vi "Disable.vi"(8 "error in (no error)":errorcluster {"code" format="%.0x"}, 11 "instrument handle":refnum<k15>) -> (0 "error out":errorcluster {"code" format="%.0x"}, 3 "instrument handle out":refnum<k15>)   [LabVIEW 2021, in "Keysight XSAnVMA.lvlib"]
doc: "Quickly places the instrument in a state where it has no, or minimal, effect on the external system to which it is connected. This state is not necessarily a known state."
uses:
  <instrlib>/Keysight XSAnVMA/Keysight XSAnVMA.lvlib
  KtXSAnVMA_64.dll
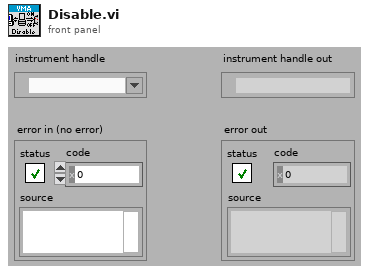
[diagram p1: front panel]
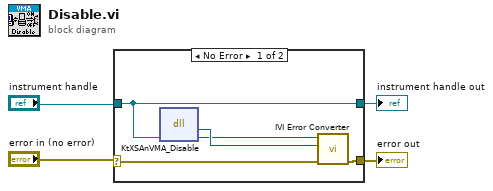
[diagram p0: block diagram]
diagram:
  n1 = case shown="No Error" "error in (no error)" {
    selector: "error in (no error)" -> [w7 w10]
    tunnel: [w9 w10] -> w4
    tunnel: "instrument handle" -> [w6 w11]
    tunnel: [w6 w11] -> w1
    frame No Error {
      n2 = dll-call lib="KtXSAnVMA**.dll" fn="KtXSAnVMA_Disable" ("LabVIEW:IviDmm_Disable")("instrument handle"=w6) -> ("Status"=w8:i32, "instrument handle"=w5:u32)  [unwired: 3 in, 2 out]
      n3 = call <instrlib>:"IVI Error Converter.vi"("error in (no error)"=w7, "IVI error code (0)"=w8, "instrument handle"=w5) -> ("error out"=w9:errorcluster)  [unwired: 7 in, 1 out]
    }
    frame Error {
    }
  }
  "error out" <- w4
  "instrument handle out" <- w1
